vi "Write Properties.vi"(8 "error in (no error)":errorcluster, 10 "Properties":map{string, T1}(c390), 11 "PropertyNode in":refnum<class "PropertyNode.lvclass">) -> (0 "error out":errorcluster, 3 "PropertyNode out":refnum<class "PropertyNode.lvclass">)   [LabVIEW 2025, in "PropertyNode.lvclass"]
uses:
  PropertyNode.lvclass
  GrowableFunctionNode.ctl
  PropertyNode.lvclass/PropertyNode.ctl
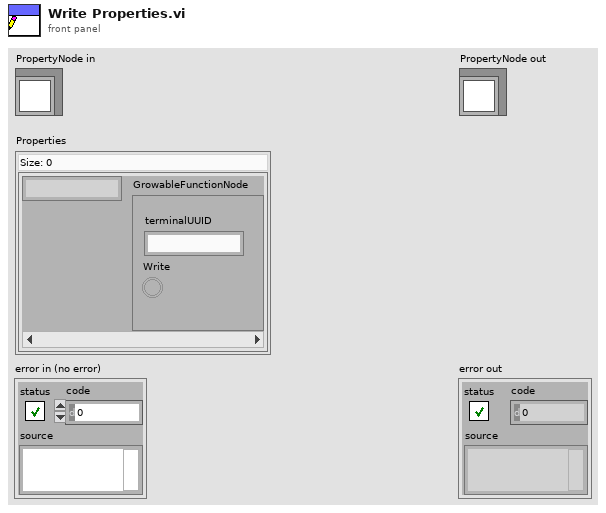
[diagram p1: front panel]
types:
  T1 = typedef "GrowableFunctionNode.ctl" = cluster{"terminalUUID":string, "Write":bool}
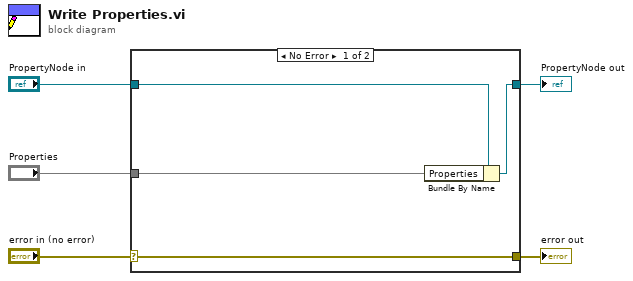
[diagram p0: block diagram]
diagram:
  n1 = case shown="No Error" "error in (no error)" {
    selector: "error in (no error)" -> [w9 w10]
    tunnel: [w9 w10] -> w4
    tunnel: [w7 w11] -> w2
    tunnel: "PropertyNode in" -> [w8 w11]
    tunnel: "Properties" -> [w6 _]
    frame No Error {
      n2 = Bundle By Name(cluster=w8, "Properties"=w6) -> (w7:refnum<class "PropertyNode.lvclass">)
    }
    frame Error {
    }
  }
  "error out" <- w4
  "PropertyNode out" <- w2
